vi "InitiateNotifiers.vi"(2 "error in (no error)":errorcluster, 3 "Boat Type":T1(ring)) -> (0 "error out":errorcluster, 1 "NotifierReferences":T2)   [LabVIEW 2013]
doc: "Initializes all the notifiers that will be used to pass data around."
uses:
  Data/TypeDefs/Notifiers.ctl
  Data/TypeDefs/UTM Location.ctl
  Data/TypeDefs/Sail Set Suggestions.ctl
  Data/TypeDefs/Rudder Set Suggestions.ctl
  Data/TypeDefs/OverrideInformation.ctl
  Data/TypeDefs/OverrideMode.ctl
  Data/TypeDefs/MotorSetup.ctl
  Data/TypeDefs/DynamixelSetupInfo.ctl
  Data/TypeDefs/AirmarStatus.ctl
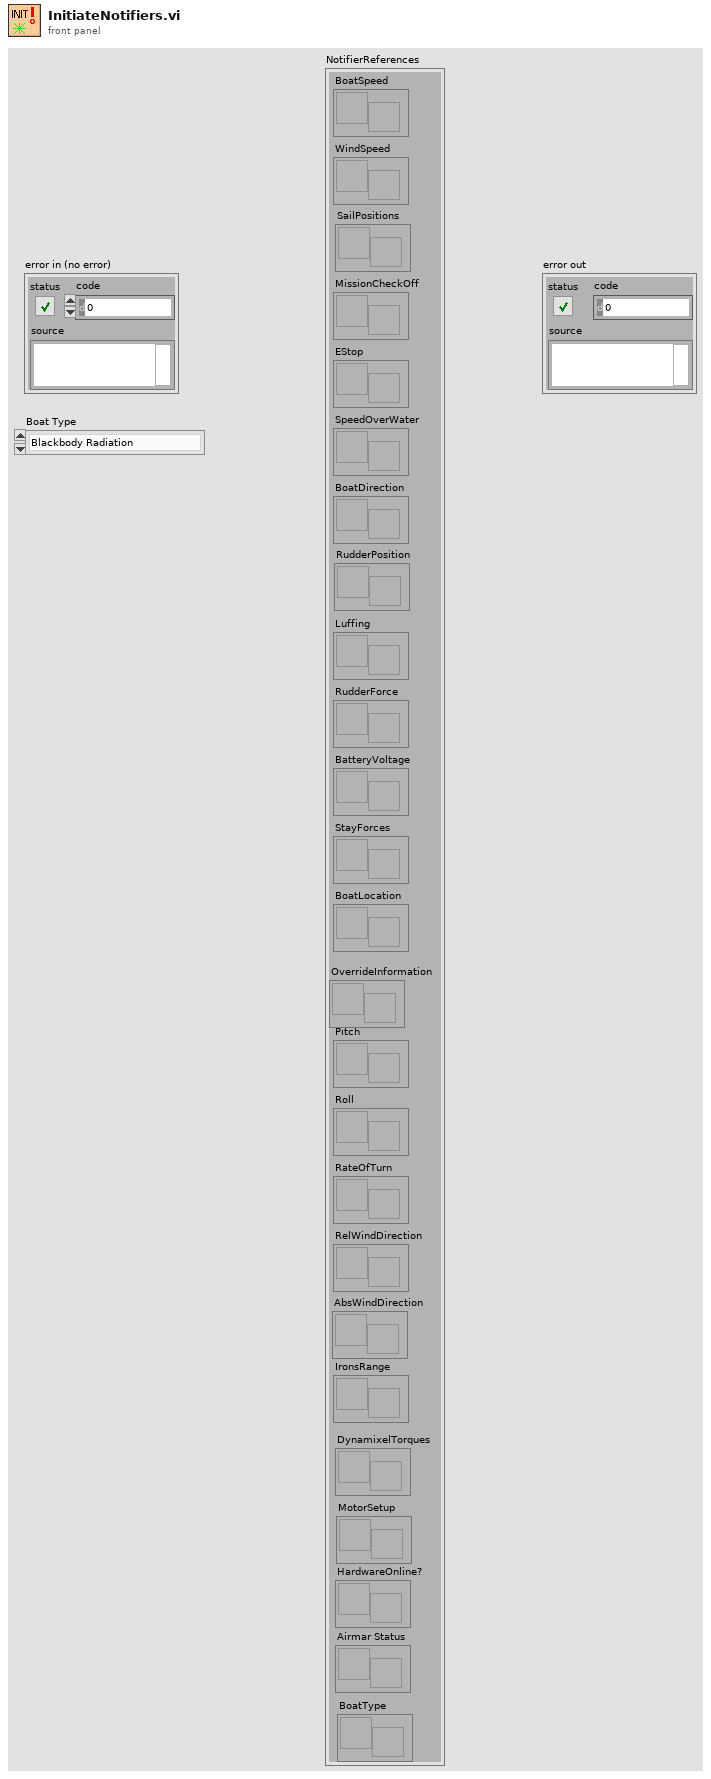
[diagram p1: front panel]
types:
  T1 = enum16{"Blackbody Radiation", "Little boats", "Simulation", "Damn Yankee"}
  T2 = typedef "Notifiers.ctl" = cluster{"BoatSpeed":refnum<notifier>, "WindSpeed":refnum<notifier>, "MissionCheckOff":refnum<notifier>, "EStop":refnum<notifier>, "SpeedOverWater":refnum<notifier>, "BoatDirection":refnum<notifier>, "Luffing":refnum<notifier>, "RudderForce":refnum<notifier>, "BatteryVoltage":refnum<notifier>, "StayForces":refnum<notifier>, "BoatLocation":refnum<notifier>, "Pitch":refnum<notifier>, "Roll":refnum<notifier>, "RateOfTurn":refnum<notifier>, "RelWindDirection":refnum<notifier>, "SailPositions":refnum<notifier>, "RudderPosition":refnum<notifier>, "IronsRange":refnum<notifier>, "AbsWindDirection":refnum<notifier>, "OverrideInformation":refnum<notifier>, "DynamixelTorques":refnum<notifier>, "HardwareOnline?":refnum<notifier>, "MotorSetup":refnum<notifier>, "Airmar Status":refnum<notifier>, "BoatType":refnum<notifier>}
  T3 = typedef "MotorSetup.ctl" = cluster{"Main Dynamixel Set Data":T4, "Rudder Dynamixel Set Data":T4, "Jib Dynamixel Set Data":T4}
  T4 = typedef "DynamixelSetupInfo.ctl" = cluster{"Lower Winch Bound":dbl, "Upper Winch Bound":dbl, "Reverse Winch Direction?":bool, "Dynamixel Cycle Number":i32}
  T5 = cluster{"AirmarOnline":bool, "WindvaneOnline":bool, "HemisphereOnline":bool, "RudderForceOnline":bool, "StayForceOnline":bool, "BatteryVoltageOnline":bool, "AccelerometerOnline":bool, "MainDynamixel Online":bool, "JibDynamixel Online":bool, "RudderDynamixel Online":bool}
  T6 = typedef "OverrideInformation.ctl" = cluster{"OverrideMode":T7, "SailSetting":T8, "Rudder Setpoint":T9}
  T7 = typedef "OverrideMode.ctl" = enum16{"None", "Rudder", "Sails", "Both"}
  T8 = typedef "Sail Set Suggestions.ctl" = cluster{"MainSailSuggestion":dbl, "JibSailSuggestion":dbl}
  T9 = typedef "Rudder Set Suggestions.ctl" = dbl
  T10 = typedef "UTM Location.ctl" = cluster{"UTM Zone":dbl, "Hemisphere":enum16{"North", "South"}, "East":dbl, "North":dbl}
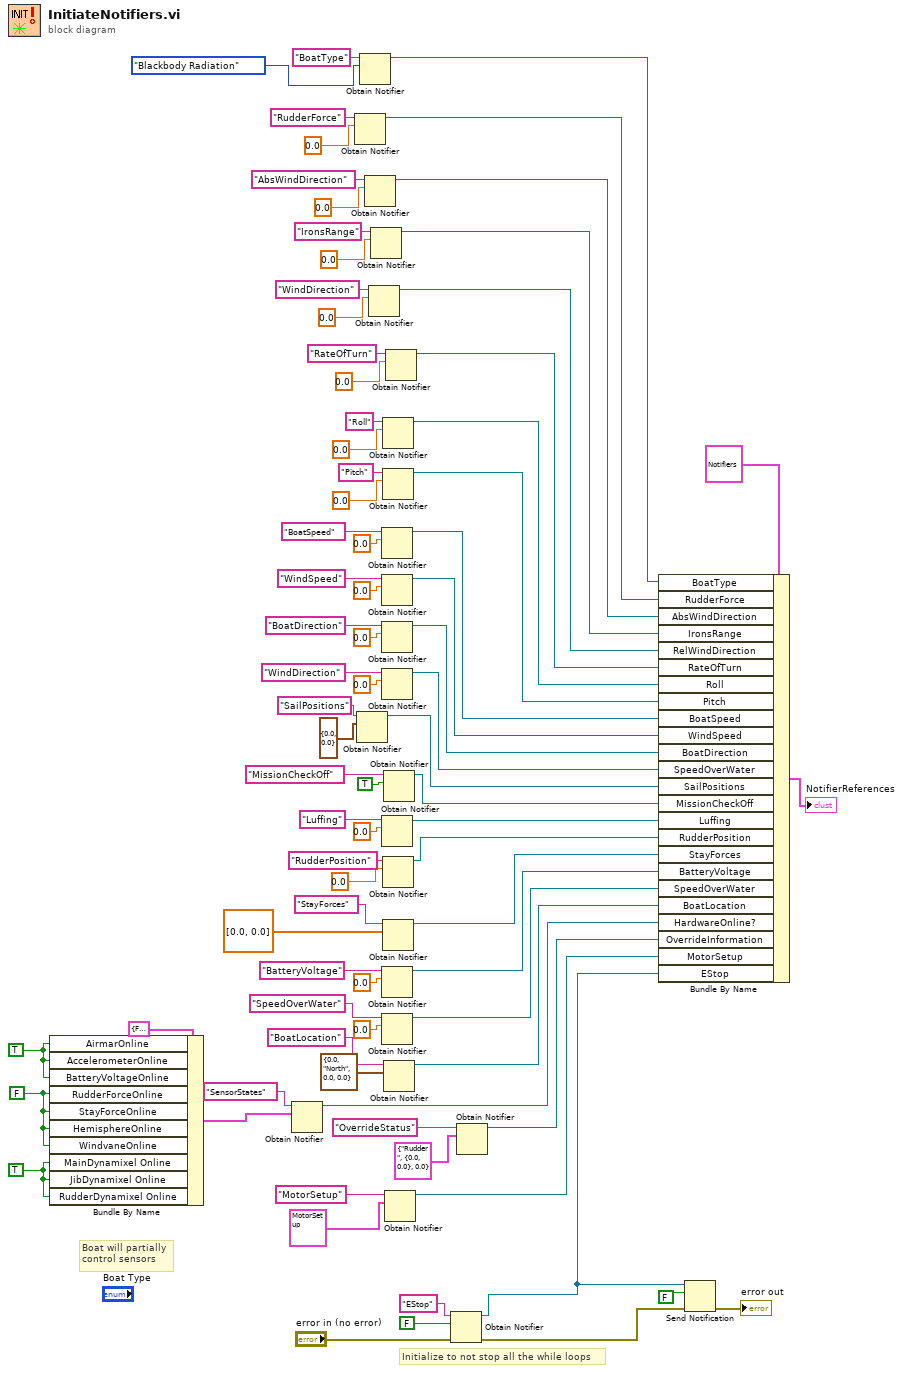
[diagram p0: block diagram]
diagram:
  w10 = TRUE
  w24 = FALSE ("AirmarOnline")
  w25 = TRUE ("AirmarOnline")
  # "Boat will partially\ncontrol sensors"
  # "Initialize to not stop all the while loops"
  n1 = Bundle By Name(cluster=T5 {"AirmarOnline"=FALSE, "WindvaneOnline"=FALSE, "HemisphereOnline"=FALSE, "RudderForceOnline"=FALSE, "StayForceOnline"=FALSE, "BatteryVoltageOnline"=FALSE, "AccelerometerOnline"=FALSE, "MainDynamixel Online"=FALSE, "JibDynamixel Online"=FALSE, "RudderDynamixel Online"=FALSE} ("latest notification"), "AirmarOnline"=w25, "AccelerometerOnline"=w25, "BatteryVoltageOnline"=w25, "RudderForceOnline"=w24, "StayForceOnline"=w24, "HemisphereOnline"=w24, "WindvaneOnline"=w24, "MainDynamixel Online"=w10, "JibDynamixel Online"=w10, "RudderDynamixel Online"=w10) -> (w23:T5)
  n2 = Obtain Notifier(name (unnamed)="SensorStates", notification data type=w23) -> (notifier out=w9:refnum<notifier>)  [unwired: 2 in, 2 out]
  n3 = Obtain Notifier(name (unnamed)="RudderForce", notification data type=0.0) -> (notifier out=w12:refnum<notifier>)  [unwired: 2 in, 2 out]
  n4 = Obtain Notifier(name (unnamed)="SailPositions", notification data type=T8 {"MainSailSuggestion"=0.0, "JibSailSuggestion"=0.0} ("output cluster")) -> (notifier out=w28:refnum<notifier>)  [unwired: 2 in, 2 out]
  n5 = Obtain Notifier(name (unnamed)="BoatType", notification data type=T1."Blackbody Radiation" ("Boat Type")) -> (notifier out=w1:refnum<notifier>)  [unwired: 2 in, 2 out]
  n6 = Obtain Notifier(name (unnamed)="AbsWindDirection", notification data type=0.0) -> (notifier out=w15:refnum<notifier>)  [unwired: 2 in, 2 out]
  n7 = Obtain Notifier(name (unnamed)="WindDirection", notification data type=0.0) -> (notifier out=w33:refnum<notifier>)  [unwired: 2 in, 2 out]
  n8 = Obtain Notifier(name (unnamed)="IronsRange", notification data type=0.0) -> (notifier out=w20:refnum<notifier>)  [unwired: 2 in, 2 out]
  n9 = Obtain Notifier(name (unnamed)="BoatSpeed", notification data type=0.0) -> (notifier out=w74:refnum<notifier>)  [unwired: 2 in, 2 out]
  n10 = Obtain Notifier(name (unnamed)="WindSpeed", notification data type=0.0) -> (notifier out=w73:refnum<notifier>)  [unwired: 2 in, 2 out]
  n11 = Obtain Notifier(name (unnamed)="BoatDirection", notification data type=0.0) -> (notifier out=w72:refnum<notifier>)  [unwired: 2 in, 2 out]
  n12 = Obtain Notifier(name (unnamed)="WindDirection", notification data type=0.0) -> (notifier out=w71:refnum<notifier>)  [unwired: 2 in, 2 out]
  n13 = Obtain Notifier(name (unnamed)="Luffing", notification data type=0.0) -> (notifier out=w55:refnum<notifier>)  [unwired: 2 in, 2 out]
  n14 = Obtain Notifier(name (unnamed)="BatteryVoltage", notification data type=0.0) -> (notifier out=w52:refnum<notifier>)  [unwired: 2 in, 2 out]
  n15 = Obtain Notifier(name (unnamed)="SpeedOverWater", notification data type=0.0) -> (notifier out=w51:refnum<notifier>)  [unwired: 2 in, 2 out]
  n16 = Obtain Notifier(name (unnamed)="Roll", notification data type=0.0) -> (notifier out=w39:refnum<notifier>)  [unwired: 2 in, 2 out]
  n17 = Obtain Notifier(name (unnamed)="Pitch", notification data type=0.0) -> (notifier out=w42:refnum<notifier>)  [unwired: 2 in, 2 out]
  n18 = Obtain Notifier(name (unnamed)="RudderPosition", notification data type=T9 0.0 ("Suggested Rudder Setpoint")) -> (notifier out=w27:refnum<notifier>)  [unwired: 2 in, 2 out]
  n19 = Obtain Notifier(name (unnamed)="StayForces", notification data type=dbl[] [0.0, 0.0] ("Array")) -> (notifier out=w53:refnum<notifier>)  [unwired: 2 in, 2 out]
  n20 = Obtain Notifier(name (unnamed)="MissionCheckOff", notification data type=TRUE) -> (notifier out=w70:refnum<notifier>)  [unwired: 2 in, 2 out]
  n21 = Obtain Notifier(name (unnamed)="BoatLocation", notification data type=T10 {"UTM Zone"=0.0, "Hemisphere"=enum."North", "East"=0.0, "North"=0.0} ("UTM Location")) -> (notifier out=w45:refnum<notifier>)  [unwired: 2 in, 2 out]
  n22 = Obtain Notifier(name (unnamed)="MotorSetup", notification data type=T3 {"Main Dynamixel Set Data"={"Lower Winch Bound"=0.0, "Upper Winch Bound"=0.0, "Reverse Winch Direction?"=FALSE, "Dynamixel Cycle Number"=0}, "Rudder Dynamixel Set Data"={"Lower Winch Bound"=0.0, "Upper Winch Bound"=0.0, "Reverse Winch Direction?"=FALSE, "Dynamixel Cycle Number"=0}, "Jib Dynamixel Set Data"={"Lower Winch Bound"=0.0, "Upper Winch Bound"=0.0, "Reverse Winch Direction?"=FALSE, "Dynamixel Cycle Number"=0}} ("latest notification")) -> (notifier out=w5:refnum<notifier>)  [unwired: 2 in, 2 out]
  n23 = Obtain Notifier(name (unnamed)="RateOfTurn", notification data type=0.0) -> (notifier out=w36:refnum<notifier>)  [unwired: 2 in, 2 out]
  n24 = Obtain Notifier(name (unnamed)="EStop", notification data type=FALSE, error in (no error)="error in (no error)") -> (notifier out=w6:refnum<notifier>, error out=w67:errorcluster)  [unwired: 1 in, 1 out]
  n25 = Obtain Notifier(name (unnamed)="OverrideStatus", notification data type=T6 {"OverrideMode"=enum."Rudder", "SailSetting"={"MainSailSuggestion"=0.0, "JibSailSuggestion"=0.0}, "Rudder Setpoint"=0.0}) -> (notifier out=w4:refnum<notifier>)  [unwired: 2 in, 2 out]
  n26 = Bundle By Name(cluster=T2 {"BoatSpeed"=refnum, "WindSpeed"=refnum, "MissionCheckOff"=refnum, "EStop"=refnum, "SpeedOverWater"=refnum, "BoatDirection"=refnum, "Luffing"=refnum, "RudderForce"=refnum, "BatteryVoltage"=refnum, "StayForces"=refnum, "BoatLocation"=refnum, "Pitch"=refnum, "Roll"=refnum, "RateOfTurn"=refnum, "RelWindDirection"=refnum, "SailPositions"=refnum, "RudderPosition"=refnum, "IronsRange"=refnum, "AbsWindDirection"=refnum, "OverrideInformation"=refnum, "DynamixelTorques"=refnum, "HardwareOnline?"=refnum, "MotorSetup"=refnum, "Airmar Status"=refnum, "BoatType"=refnum} ("NotifierReff 2"), "BoatType"=w1, "RudderForce"=w12, "AbsWindDirection"=w15, "IronsRange"=w20, "RelWindDirection"=w33, "RateOfTurn"=w36, "Roll"=w39, "Pitch"=w42, "BoatSpeed"=w74, "WindSpeed"=w73, "BoatDirection"=w72, "SpeedOverWater"=w71, "SailPositions"=w28, "MissionCheckOff"=w70, "Luffing"=w55, "RudderPosition"=w27, "StayForces"=w53, "BatteryVoltage"=w52, "SpeedOverWater"=w51, "BoatLocation"=w45, "HardwareOnline?"=w9, "OverrideInformation"=w4, "MotorSetup"=w5, "EStop"=w6) -> (→"NotifierReferences":T2)
  n27 = Send Notification(notification=FALSE, notifier=w6, error in (no error)=w67) -> (error out=→"error out":errorcluster)  [unwired: 1 out]
